vi "SaveDataArray.vi"(5 "Lane_Number":string(combo)="ST1_", 7 "Name_Test":string(combo)="D_L_", 8 "VoltArray1":dbl[](array[numeric]), 9 "VoltArray":dbl[](array[numeric]), 10 "ForceArray":dbl[](array[numeric]), 11 "StockArray":dbl[](array[numeric])) -> ()   [LabVIEW 2017]
uses:
  <vilib>/Utility/file.llb/Write Delimited Spreadsheet (string).vi
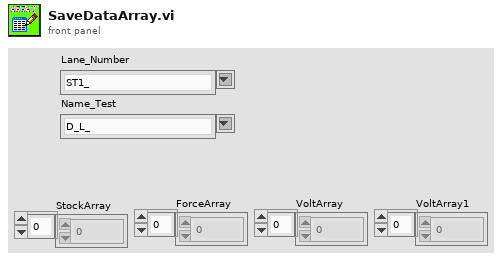
[diagram p1: front panel]
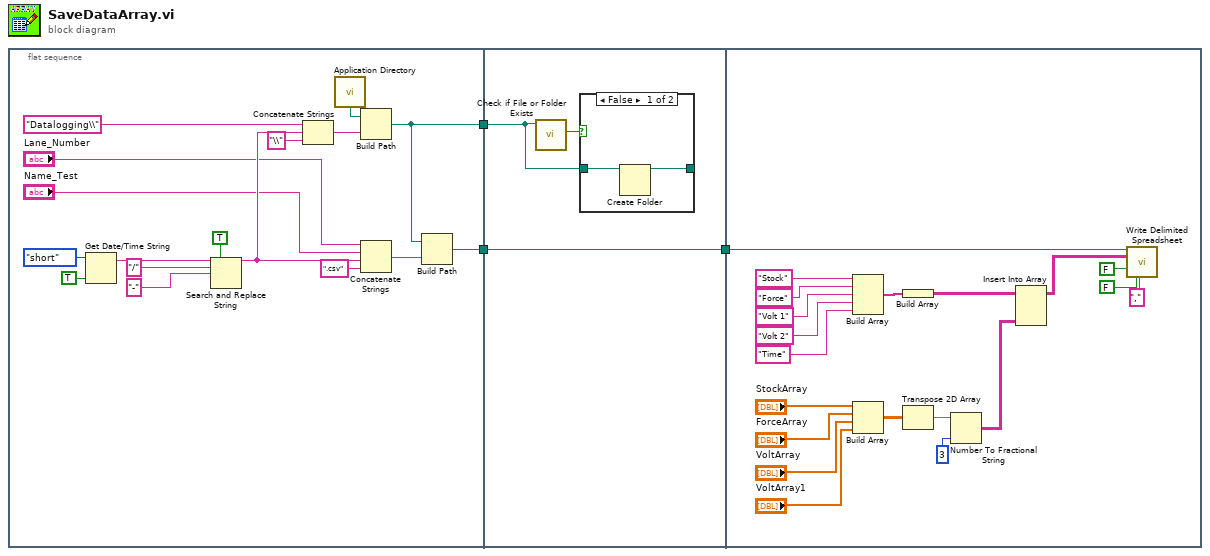
[diagram p0: block diagram]
diagram:
  n1 = flat-sequence {
    tunnel: [w11] -> w3
    tunnel: [w10] -> w2
    tunnel: w3 -> [w22]
    tunnel: [w21] -> w1
    tunnel: w2 -> [w21]
    tunnel: w1 -> [w46]
    frame #0 {
      n2 = Get Date/Time String(date format (0)=enum16{"short", "long", "abbreviated"}."short", want seconds? (F)=TRUE) -> (date string=w7:string)  [unwired: 1 in, 1 out]
      n3 = Search and Replace String(replace all?=TRUE ("replace all? (F)"), input string=w7, search string="/" ("input string"), replace string="-" ("replace string (\"\")")) -> (result string=w15:string)  [unwired: 4 in, 3 out]
      n4 = Concatenate Strings("Datalogging\\", w15, "\\" ("string")) -> (w12:string)
      n5 = call <vilib>:"Application Directory.vi"() -> ("Application Directory"=w13:path)
      n6 = Build Path(base path=w13, name or relative path=w12) -> (appended path=w11:path)
      n7 = Concatenate Strings("Lane_Number", "Name_Test", w15, ".csv" ("string")) -> (w17:string)
      n8 = Build Path(base path=w11, name or relative path=w17) -> (appended path=w10:path)
    }
    frame #1 {
      n9 = call <vilib>:"Check if File or Folder Exists.vi"("path"=w22) -> ("file or folder exists?"=w23:bool)  [unwired: 8 in, 2 out]
      n10 = case shown="False" w23 {
        tunnel: w22 -> [w25 w26]
        tunnel: [w24 w26] -> _
        frame False {
          n11 = Create Folder(path (use dialog)=w25) -> (created path=w24:path)  [unwired: 2 in, 2 out]
        }
        frame True {
        }
      }
    }
    frame #2 {
      n12 = Build Array("Stock", "Force", "Volt 1", "Volt 2", "Time") -> (w43:string[])
      n13 = Build Array("StockArray", "ForceArray", "VoltArray", "VoltArray1") -> (w32:dbl[][])
      n14 = Build Array(w43) -> (w30:string[][])
      n15 = Transpose 2D Array(2D array=w32) -> (transposed array=w31:dbl[][])
      n16 = Number To Fractional String(number=w31, precision (6)=i16 3) -> (F-format string=w29:string[][])  [unwired: 2 in]
      n17 = Insert Into Array(array=w30, new element=w29) -> (w28:string[][])  [unwired: 2 in]
      n18 = call-poly <vilib>:"Write Delimited Spreadsheet.vi"("file path (dialog if empty)"=w46, "2D data"=w28, "append to file? (new file:F)"=FALSE, "transpose? (no:F)"=FALSE, "delimiter (\\t)"="," ("delimiter (\\t)")) -> ()  [unwired: 9 in, 2 out]
    }
  }
